vi "bin_counts.vi"(8 "#clock cycles":i32=10000, 9 "#bins":u32=10, 10 "counter timetag list":u32[](array[numeric])) -> (0 "cycles per bin":u32=10, 1 "bins":dbl[](array[numeric]), 2 "#counts":u32=10, 3 "histogram":i32[](array[numeric]))   [LabVIEW 2018]
uses:
  <vilib>/Analysis/1siggen.llb/Ramp Pattern by Samples.vi
  <vilib>/Analysis/NI_AALBase.lvlib
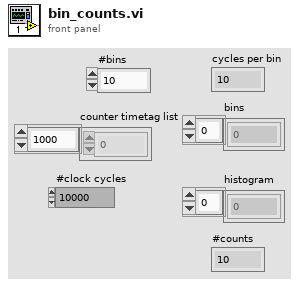
[diagram p1: front panel]
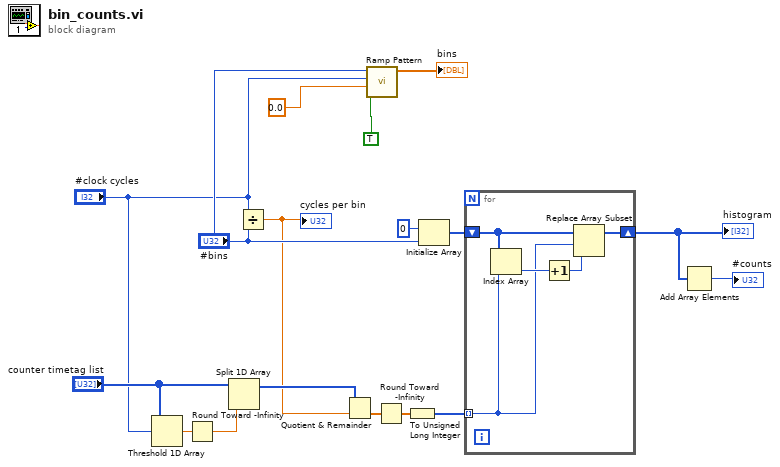
[diagram p0: block diagram]
diagram:
  n1 = Threshold 1D Array(2:"#clock cycles", 3:"counter timetag list") -> (0:w17:dbl)  [unwired: 1 in]
  n2 = Round Toward -Infinity(1:w17) -> (0:w16:dbl)
  n3 = Split 1D Array(array="counter timetag list", index=w16) -> (first subarray=w12:u32[])  [unwired: 1 out]
  n4 = Divide(x="#clock cycles", y="#bins") -> (x/y=w3:dbl)
  "cycles per bin" <- w3
  n5 = Quotient & Remainder(x=w12, y=w3) -> (floor(x/y)=w13:dbl[])  [unwired: 1 out]
  n6 = call-poly <vilib>:"Ramp Pattern.vi"("exclude end?"=TRUE, "start"=0.0, "end"="#clock cycles", "samples"="#bins") -> ("Ramp Pattern"=→"bins":dbl[])  [unwired: 6 in, 1 out]
  n7 = Round Toward -Infinity(1:w13) -> (0:w14:dbl[])
  n8 = To Unsigned Long Integer(number=w14) -> (unsigned 32bit integer=w11:u32[])
  n9 = Initialize Array(u32 0 ("element"), "#bins") -> (w10:u32[])
  n10 = for {
    shift-right: [w22] -> w2
    shift-left: w10 -> [w21]
    tunnel: w11 -> [w18] mode=indexing
    n11 = Index Array(array=w21, index=w18) -> (element=w20:u32)
    n12 = Increment(x=w20) -> (x+1=w19:u32)
    n13 = Replace Array Subset(array=w21, new element=w19, index=w18) -> (w22:u32[])
  }
  "histogram" <- w2
  n14 = Add Array Elements(numeric array=w2) -> (sum=→"#counts":u32)
